vi "ATI_Request.vi"(8 "error in (no error)":errorcluster, 10 "Command":string, 11 "VISA resource name":refnum<visa-resource-name>="Master_Oscilloscope") -> (0 "error out":errorcluster, 1 "read buffer":string, 2 "Active?":bool, 3 "VISA resource name out":refnum<visa-resource-name>)   [LabVIEW 2020]
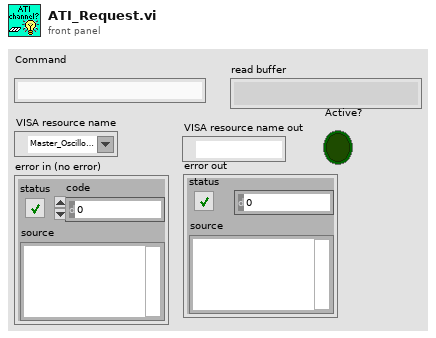
[diagram p1: front panel]
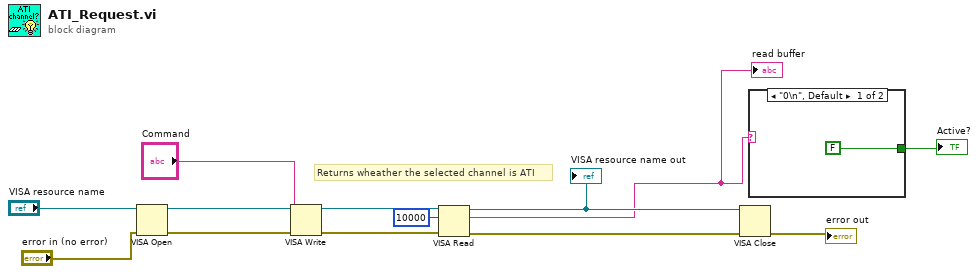
[diagram p0: block diagram]
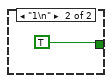
[diagram p2: hidden frame]
diagram:
  # "Returns wheather the selected channel is ATI"
  n1 = VISA Open(error in (no error)="error in (no error)", VISA resource name="VISA resource name") -> (VISA resource name=w6:refnum<visa-resource-name>, error out=w4:errorcluster)  [unwired: 3 in]
  n2 = VISA Write(VISA resource name=w6, write buffer="Command", error in (no error)=w4) -> (VISA resource name out=w13:refnum<visa-resource-name>, error out=w12:errorcluster)  [unwired: 1 out]
  n3 = VISA Read(VISA resource name=w13, byte count=u32 10000, error in (no error)=w12) -> (VISA resource name out=w10:refnum<visa-resource-name>, read buffer=w3:string, error out=w9:errorcluster)  [unwired: 1 out]
  "VISA resource name out" <- w10
  "read buffer" <- w3
  n4 = VISA Close(VISA resource name=w10, error in (no error)=w9) -> (error out=→"error out":errorcluster)
  n5 = case shown="\"0\\n\", Default" w3 {
    tunnel: [FALSE TRUE] -> w2
    frame "0\n", Default {
    }
    frame "1\n" {
    }
  }
  "Active?" <- w2
